vi "Timer_Reset.vi"(8 "error in (no error)":errorcluster, 11 "Timer Data Reference (in)":refnum<data-value>) -> (0 "error out":errorcluster, 3 "Timer Data Reference (out)":refnum<data-value>)   [LabVIEW 2024]
doc: "Resets the Timer DVR\n\n--------\nPaulo Rossi\nprossi@aurumautomation.ca\n©2024 Aurum Automation Inc.\nOpen-Sourced per GNU GPL v3\n\nYou should have received a copy of the GNU General Public License along with this program. If not, see <https://www.gnu.org/licenses/>.s"
uses:
  Timer_Data.ctl
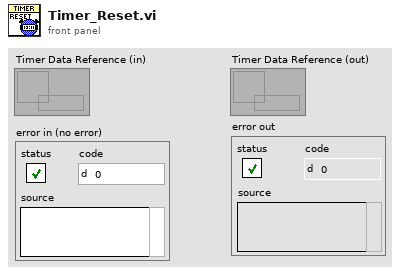
[diagram p1: front panel]
types:
  T1 = typedef "Timer_Data.ctl" = cluster{"Starting Time":dbl, "Time Elapsed (s)":dbl, "Is Time Elapsed?":bool, "Target Time (s)":dbl, "Pause Start Time":dbl, "Pause Elapsed Time":dbl, "Is Paused?":bool, "Cumulative Paused Time":dbl}
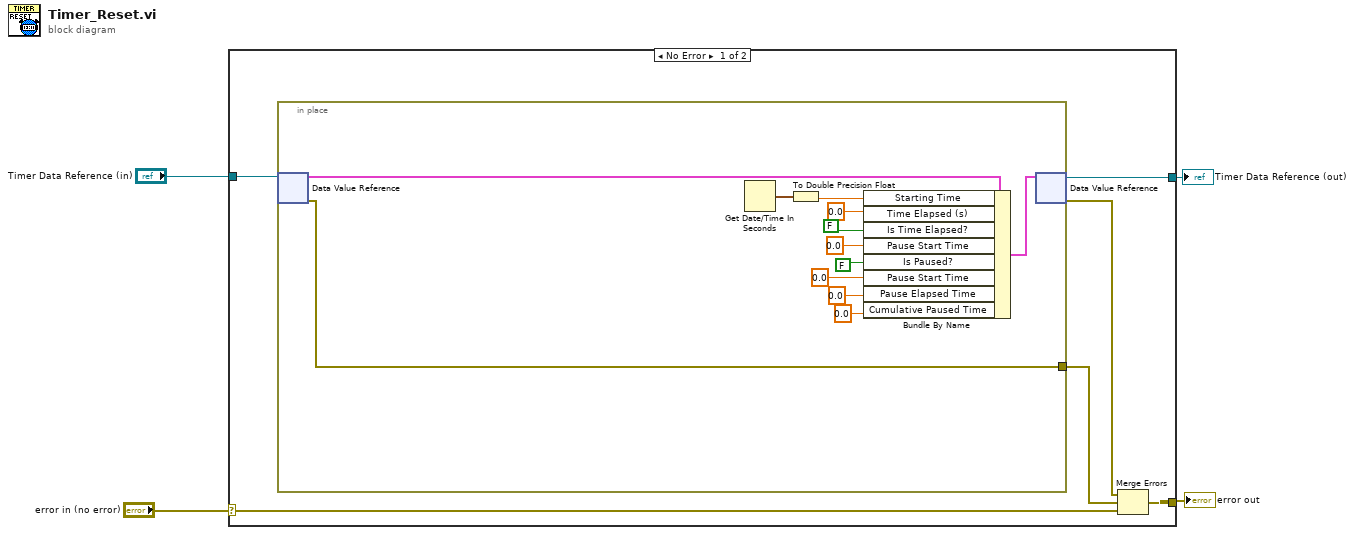
[diagram p0: block diagram]
diagram:
  n1 = case shown="No Error" "error in (no error)" {
    selector: "error in (no error)" -> [w5 w24]
    tunnel: [w8 w24] -> w3
    tunnel: "Timer Data Reference (in)" -> [w10 w23]
    tunnel: [w9 w23] -> w1
    frame No Error {
      n2 = in-place {
        in-place-border: [w21] -> w6
        n3 = in-place-dvr #1(w10) -> (w20:T1, w21:errorcluster)
        n4 = Get Date/Time In Seconds() -> (seconds since 1Jan1904=w15:timestamp)
        n5 = To Double Precision Float(number=w15) -> (double precision float=w14:dbl)
        n6 = Bundle By Name(cluster=w20, "Starting Time"=w14, "Time Elapsed (s)"=0.0, "Is Time Elapsed?"=FALSE ("Is Paused?"), "Pause Start Time"=0.0 ("Pause Elapsed Time"), "Is Paused?"=FALSE, "Pause Start Time"=0.0, "Pause Elapsed Time"=0.0, "Cumulative Paused Time"=0.0) -> (w22:T1)
        n7 = in-place-dvr #1(w22) -> (w9:refnum<data-value>, w7:errorcluster)
      }
      n8 = Merge Errors(w7, w6, w5) -> (w8:errorcluster)
    }
    frame Error {
    }
  }
  "error out" <- w3
  "Timer Data Reference (out)" <- w1
